vi "GCMPlugin_IsSupportingItem.vi"(8 "error in (no error)":errorcluster, 9 "VI Reference":refnum<vi>, 10 "ProjectItem Refnum":refnum<vi>, 11 "_BasicVIDocumentation in":refnum<class "GCMIconEditor.lvclass">) -> (0 "error out":errorcluster, 2 "IsSupportingItem":bool, 3 "_BasicVIDocumentation out":refnum<class "GCMIconEditor.lvclass">)   [LabVIEW 2014, in "GCMIconEditor.lvlib" / "GCMIconEditor.lvclass"]
uses:
  GCMIconEditor.lvclass
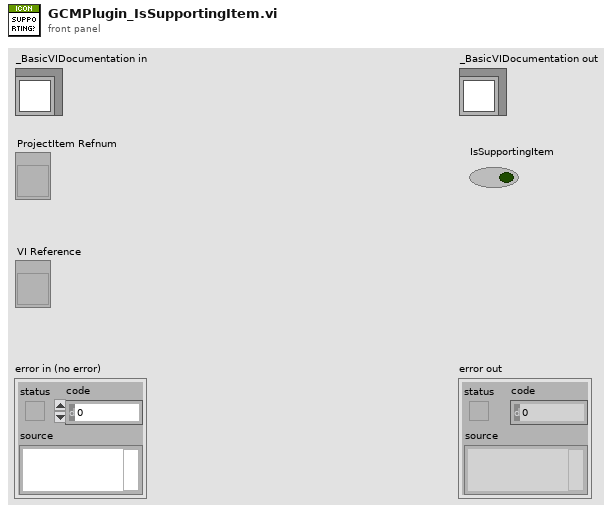
[diagram p1: front panel]
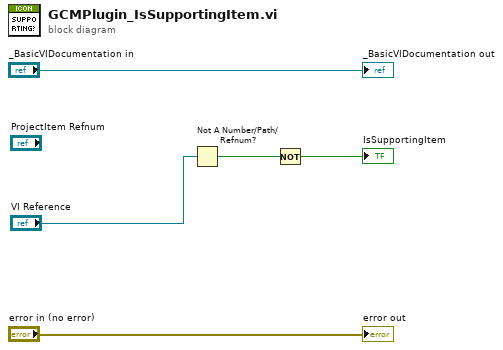
[diagram p0: block diagram]
diagram:
  n1 = Not A Number/Path/Refnum?(number/path/refnum="VI Reference") -> (NaN/Path/Refnum?=w2:bool)
  n2 = Not(x=w2) -> (.not. x?=→"IsSupportingItem":bool)
  "error out" <- "error in (no error)"
  "_BasicVIDocumentation out" <- "_BasicVIDocumentation in"
